vi "Test Panel - Single Loop.vi"(8 "Error in":errorcluster, 9 "TDMS Name Mapping":T5={"FGEN Channel Mapping"=[["0", "Chn0"]], "DAQ Channel Mapping"=[["port0/line1", "PA ON"], ["port0/line2", "Gate IN"], ["port0/line3", "Damping"], ["port0/line4", "Rx ON"]], "FGEN Wfm List"=[["Wfm1", "FGEN_Wfm1"], ["Wfm2", "FGEN_Wfm2"]], "DAQ Wfm List"=[["Wfm1", "DAQ_Wfm1"], ["Wfm2", "DAQ_Wfm2"]]}, 10 "Wavefom Sequence":T4={"FGEN Wfm Sequence"=["Wfm1"], "DAQ Wfm Sequence"=["Wfm1"], "Loops"=[1]}, 11 "Resource Settings":T3={"FGEN Resource"="", "DAQmx Resource"="", "TDMS File Path"=path "", "Scope Resource"="", "Scope Config File Path"=path "", "Trigger Delay"=0.0, "Duration"=-1.0, "Fetch Timeout"=5.0} {"Fetch Timeout" format="%#.5ps"; "Duration" format="%#_6ps"; "Trigger Delay" format="%#_gs"}) -> (0 "Error out":errorcluster, 1 "FFT Waveforms (dB)":T7(graph), 2 "FFT Waveforms (Volt RMS)":T7(graph), 3 "Time Domain Waveforms":T7(graph), 4 "Scope Result Ctrl Refs Out":T8)   [LabVIEW 2025]
uses:
  Live Graph Plotter/Live Graph Plotter.lvclass
  <extravilib>/ChannelInstances/Tag-bool.lvlib
  Typedef/Scope Result Ctrl Refs.ctl
  Typedef/TDMS Name Mapping.ctl
  Typedef/Resource Settings.ctl
panel:
  out "Actual Sample Rates":T1 {"FGEN Sample Rate" format="%#_6pHz"; "DAQ Sample Rate" format="%#_6pHz"; "SCOPE Sample Rate" format="%#_6pHz"}
  in  "Stop":bool
  in  "Tab Control":T2(tab)
  in  "Results":T6(tab)
  # "FGEN - Scope - Digital DAQ Test Panel (Single Loop)"
  # "Right-click the graph to export waveforms to file"
  # "* Negative duration will keep the original waveform length in the scope settings"
  # "* Make sure the number of elements in each array are match"
  # "This Test Panel can control FGEN and DAQ to generate a sequence of analog and \ndigital waveforms from a TDMS file. While generating, it can also control SCOPE to \ncapture multiple records according to the number of steps in the Waveform \nSequence (FGEN or DAQ).\n\nYou can choose to disable FGEN, DAQ or SCOPE function by leaving thier Resource \nNames blank. \n\nIf FGEN and DAQ are enabled, DAQ will arm the FGEN start trigger before it starts \ngeneration through the PXI backplane (implicit triggering). If only DAQ enabled,\nDAQ will start generation immediately.\n\nBefore start, prepare a TMDS waveform file that matches the TDMS Name Mapping:\n  - For FGEN:\n      - Refer to the FGEN Channel Mapping and FGEN Wfm List.\n      - FGEN will run with the Arbitrary Sequence mode and Single Trigger mode to \n         generate the waveforms in the FGEN Wfm Sequence. \n      - Data will resampled to the highest sample rate among all the FGEN waveforms.\n  - For DAQ:\n     - Refer to the DAQ Channel Mapping and DAQ Wfm List\n     - The waveforms specified in the DAQ Wfm Sequence will be cascaded as one \n        waveform for each channel. \n     - Data will resampled to the highest sample rate among all the DAQ waveforms.\n\nThen, configure the FGEN and DAQ Sequence accordingly. By default, each step \nonly loops once. You can increase it to more. The number  of records to be captured \nby SCOPE will be total number of loops. You must make sure the number of \nsequence steps and loops are equal. The code doesn't check the consistency.  \n\nUse the InstrumentStudio to configure the settings of SCOPE first, and export the \nsettings as .niscopeconfig file. Then, you can use the file to configure the settings\nin this Test Panel."
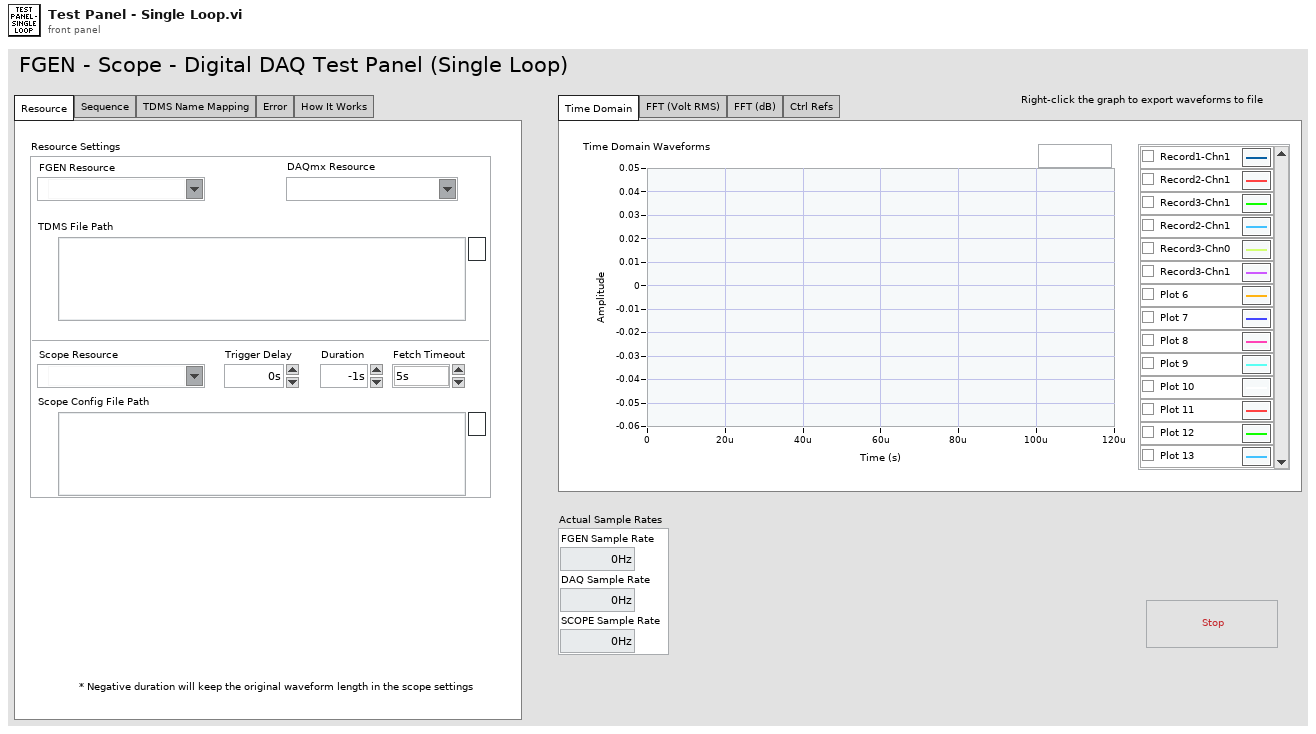
[diagram p1: front panel]
types:
  T1 = cluster{"FGEN Sample Rate":dbl, "DAQ Sample Rate":dbl, "SCOPE Sample Rate":dbl}
  T2 = enum32{"Resource", "Sequence", "TDMS Name Mapping", "Error", "How It Works"}
  T3 = typedef "Resource Settings.ctl" = cluster{"FGEN Resource":refnum<k15>, "DAQmx Resource":tag, "TDMS File Path":path, "Scope Resource":refnum<k15>, "Scope Config File Path":path, "Trigger Delay":dbl, "Duration":dbl, "Fetch Timeout":dbl}
  T4 = cluster{"FGEN Wfm Sequence":string[], "DAQ Wfm Sequence":string[], "Loops":i32[]}
  T5 = typedef "TDMS Name Mapping.ctl" = cluster{"FGEN Channel Mapping":string[][], "DAQ Channel Mapping":string[][], "FGEN Wfm List":string[][], "DAQ Wfm List":string[][]}
  T6 = enum32{"Time Domain", "FFT (Volt RMS)", "FFT (dB)", "Ctrl Refs"}
  T7 = cluster{"relativeInitialX":dbl, "xIncrement":dbl, "wfm":dbl[]}[]
  T8 = typedef "Scope Result Ctrl Refs.ctl" = cluster{"Time Waveforms Graph Ref":refnum<class "Live Graph Plotter.lvclass">, "FFT Volt RMS Graph Ref":refnum<class "Live Graph Plotter.lvclass">, "FFT dB Graph Ref":refnum<class "Live Graph Plotter.lvclass">}
  T9 = typedef "Test Panel State Data.ctl" = cluster{"FGEN Resource":refnum<k15>, "DAQmx Tasks Session":cluster{"DO Task":refnum<k21>, "Ctr0 Task":refnum<k21>}, "Scope Resource":refnum<k15>, "FGEN Enabled?":bool, "DAQ Enabled?":bool, "Scope Enabled?":bool, "Max Total FGEN Wfm Duration (s)":dbl, "FGEN-DAQ Routing":cluster{"FGEN Start Trigger":string, "DAQ Trig Line":string}, "Scope Recording Settings":T10}
  T10 = typedef "Scope Recording Settings.ctl" = cluster{"Number of Records":i32, "Channels Per Record":i32, "Plot Names":string[][], "Fetch Timeout":dbl, "Channel List":string}
  T11 = typedef "Tag-bool.lvlib/))Channel.ctl" = refnum<queue>
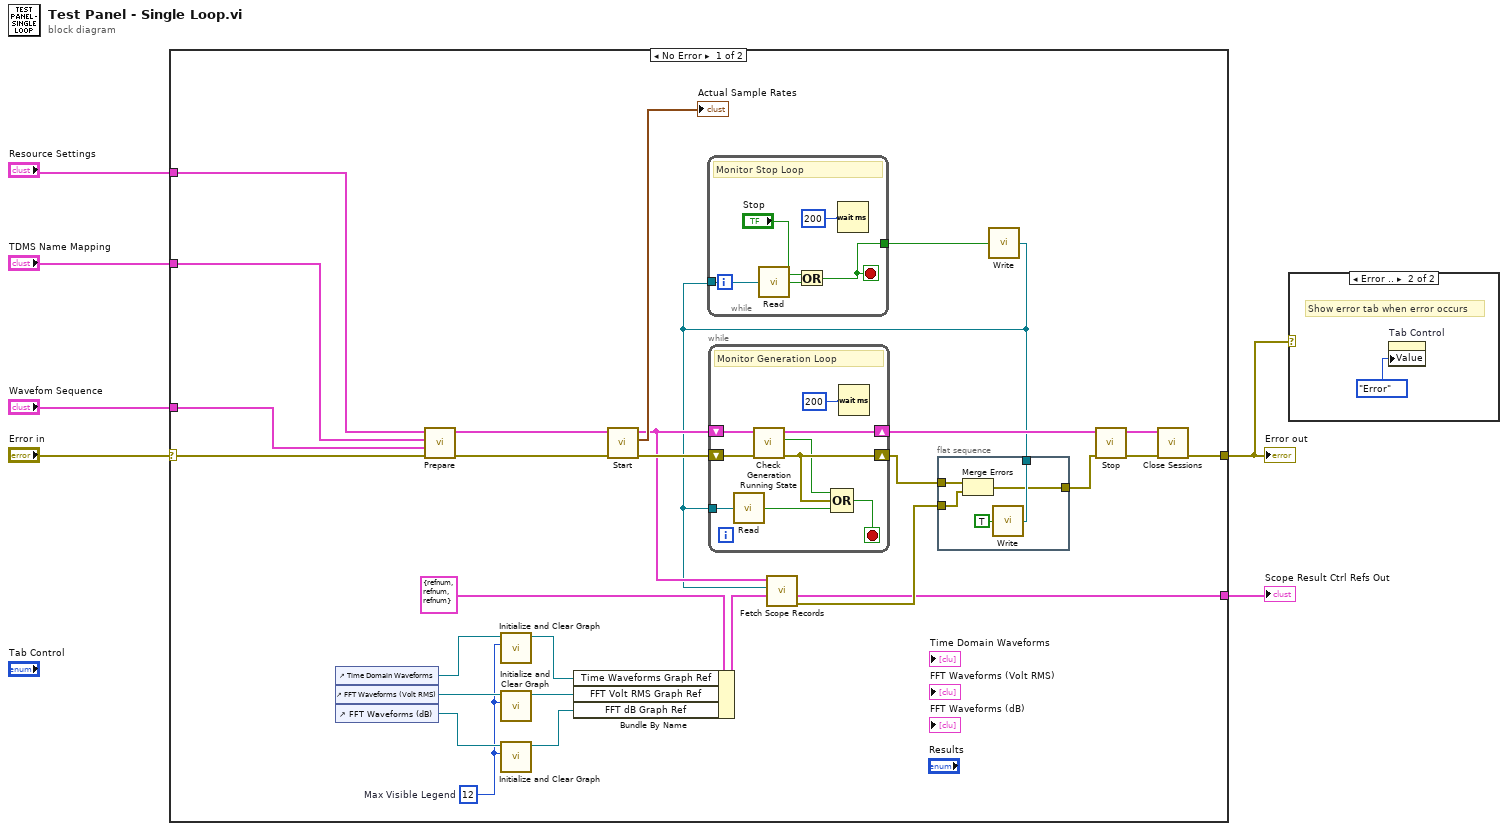
[diagram p0: block diagram]
diagram:
  n1 = case shown="No Error" "Error in" {
    selector: "Error in" -> [w31 w54]
    tunnel: [w9 w54] -> w3
    tunnel: "Resource Settings" -> [w34 _]
    tunnel: "TDMS Name Mapping" -> [w33 _]
    tunnel: "Wavefom Sequence" -> [w32 _]
    tunnel: [w7 _] -> w1
    frame No Error {
      w10 = 12  # Max Visible Legend
      n2 = control-ref of="Time Domain Waveforms"() -> (w16:refnum<vi>)
      n3 = control-ref of="FFT Waveforms (Volt RMS)"() -> (w15:refnum<vi>)
      n4 = control-ref of="FFT Waveforms (dB)"() -> (w11:refnum<vi>)
      n5 = call "Prepare.vi"("error in (no error)"=w31, "Wavefom Sequence"=w32, "TDMS Name Mapping"=w33, "Resource Settings"=w34) -> ("error out"=w30:errorcluster, "Panel State Data Out"=w29:T9)  [unwired: 6 in]
      n6 = call "Initialize and Clear Graph.vi"("Max Visible Legend"=w10, "WaveformGraph Ref"=w16) -> ("Live Graph Plotter out"=w14:refnum<class "Live Graph Plotter.lvclass">)  [unwired: 8 in, 1 out]
      n7 = call "Initialize and Clear Graph.vi"("Max Visible Legend"=w10, "WaveformGraph Ref"=w15) -> ("Live Graph Plotter out"=w13:refnum<class "Live Graph Plotter.lvclass">)  [unwired: 8 in, 1 out]
      n8 = call "Initialize and Clear Graph.vi"("Max Visible Legend"=w10, "WaveformGraph Ref"=w11) -> ("Live Graph Plotter out"=w12:refnum<class "Live Graph Plotter.lvclass">)  [unwired: 8 in, 1 out]
      n9 = Bundle By Name(cluster=T8 {"Time Waveforms Graph Ref"=refnum, "FFT Volt RMS Graph Ref"=refnum, "FFT dB Graph Ref"=refnum} ("Scope Result Ctrl Refs"), "Time Waveforms Graph Ref"=w14, "FFT Volt RMS Graph Ref"=w13, "FFT dB Graph Ref"=w12) -> (w17:T8)
      n10 = call "Start.vi"("error in (no error)"=w30, "Panel State Data In"=w29) -> ("error out"=w26:errorcluster, "Actual Sample Rates"=→"Actual Sample Rates":T1, "Panel State Data Out"=w24:T9)  [unwired: 7 in]
      n11 = flat-sequence {
        tunnel: w22 -> [w39]
        tunnel: w21 -> [w38]
        tunnel: w20 -> [w36]
        tunnel: [w35] -> w19
        frame #0 {
          n12 = Merge Errors(w39, w38) -> (w35:errorcluster)
          n13 = call <extravilib>:"Write.vi"("element"=TRUE) -> ("channel"=w36:T11)  [unwired: 1 out]
        }
      }
      n14 = while {
        tunnel: [w51] -> w25
        tunnel: w20 -> [w50]
        stop <- w51 stop-if-true
        # "Monitor Stop Loop"
        n15 = call <extravilib>:"Read.vi"("channel"=w50) -> ("element"=w49:bool)  [unwired: 1 in, 1 out]
        n16 = Or(x="Stop", y=w49) -> (x .or. y?=w51:bool)
        n17 = Wait (ms)(milliseconds to wait=u32 200) -> ()  [unwired: 1 out]
      }
      n18 = call <extravilib>:"Write.vi"("element"=w25) -> ("channel"=w20:T11)  [unwired: 1 out]
      n19 = while {
        shift-right: [w45] -> w22
        shift-left: w26 -> [w48]
        shift-right: [w44] -> w23
        shift-left: w24 -> [w47]
        tunnel: w20 -> [w41]
        stop <- w46 stop-if-true
        # "Monitor Generation Loop"
        n20 = call <extravilib>:"Read.vi"("channel"=w41) -> ("element"=w40:bool)  [unwired: 1 in, 1 out]
        n21 = call "Check Generation Running State.vi"("error in (no error)"=w48, "Panel State Data In"=w47) -> ("error out"=w45:errorcluster, "Is Done?"=w42:bool, "Panel State Data Out"=w44:T9)  [unwired: 7 in]
        n22 = Compound Arithmetic op=OR(w42, w45, w40) -> (w46:bool)
        n23 = Wait (ms)(milliseconds to wait=u32 200) -> ()  [unwired: 1 out]
      }
      n24 = call "Fetch Scope Records.vi"("Scope Result Ctrl Refs In"=w17, "Stop Channel"=w20, "Panel State Data In"=w24) -> ("error out"=w21:errorcluster, "Scope Result Ctrl Refs Out"=w7:T8)  [unwired: 6 in, 1 out]
      n25 = call "Stop.vi"("error in (no error)"=w19, "Panel State Data In"=w23) -> ("error out"=w28:errorcluster, "Panel State Data Out"=w8:T9)  [unwired: 8 in]
      n26 = call "Close Sessions.vi"("error in (no error)"=w28, "Panel State Data In"=w8) -> ("error out"=w9:errorcluster)  [unwired: 8 in, 1 out]
    }
    frame Error {
    }
  }
  "Error out" <- w3
  "Scope Result Ctrl Refs Out" <- w1
  n27 = case shown="Error .." w3 {
    frame No Error {
    }
    frame Error {
      # "Show error tab when error occurs"
      n28 = property on="Tab Control" class="TabCtl (strict)"("Value"=T2."Error" ("Tab Control")) -> ()  [unwired: 2 in, 2 out]
    }
  }
